vi "Calc - P2.vi"(10 "P1":dbl, 11 "PODF":dbl) -> (3 "P2":dbl)   [LabVIEW 2018, in "Controller (Host).lvlib"]
uses:
  Controller (Host).lvlib
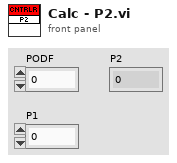
[diagram p1: front panel]
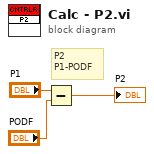
[diagram p0: block diagram]
diagram:
  # "P2\nP1-PODF"
  n1 = Subtract(x="P1", y="PODF") -> (x-y=→"P2":dbl)
